vi "Read Multi Eval Meas Phase Error Results.vi"(8 "error in (no error)":errorcluster, 9 "Result Type (Current)":i32(ring) items=["Current"=0, "Average"=1, "Maximum"=4], 10 "Instance (1)":T1=1, 11 "VISA resource name":refnum<visa-resource-name>) -> (0 "error out":errorcluster, 1 "Phase Error Results":cluster{"Low":dbl, "High":dbl}[](array[cluster]) {"High" format="%^.3e"; "Low" format="%^.3e"}, 2 "Reliability":i32, 3 "VISA resource name out":refnum<visa-resource-name>)   [LabVIEW 2015, in "Rohde&Schwarz CMXP NR FR2 Measurement.lvlib"]
doc: "Starts a new single shot measurement and returns the multi eval measurement values of the phase error bar graphs for the OFDM symbols in the measured slot.\n\nAttributes:\nRSCMXPNRFR2M_ATTR_READ_MULTI_EVAL_MEASUREMENT_PERR_AVERAGE_RESULTS\nRSCMXPNRFR2M_ATTR_READ_MULTI_EVAL_MEASUREMENT_PERR_CURRENT_RESULTS\nRSCMXPNRFR2M_ATTR_READ_MULTI_EVAL_MEASUREMENT_PERR_MAXIMUM_RESULTS\n\nRemote-control commands:\nREAD:NRMMw:MEAS<i>:MEValuation:PERRor:AVERage?\nREAD:NRMMw:MEAS<i>:MEValuation:PERRor:CURRent?\nREAD:NRMMw:MEAS<i>:MEValuation:PERRor:MAXimum?"
uses:
  <instrlib>/Rohde&Schwarz CMXP NR FR2 Measurement/Rohde&Schwarz CMXP NR FR2 Measurement.lvlib
  <instrlib>/Rohde&Schwarz CMXP NR FR2 Measurement/Private/_Instance.ctl
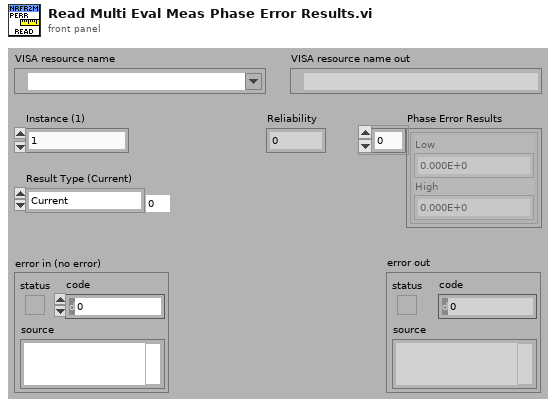
[diagram p1: front panel]
types:
  T1 = typedef "Rohde&Schwarz CMXP NR FR2 Measurement.lvlib/_Instance.ctl" = i32
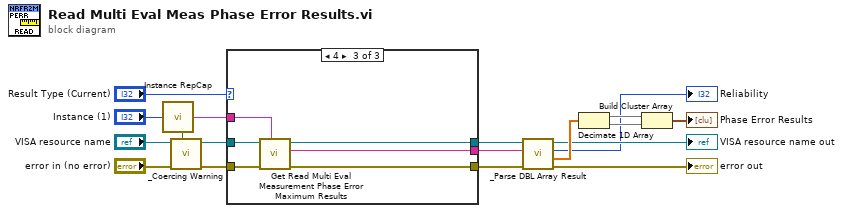
[diagram p0: block diagram]
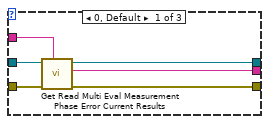
[diagram p2: hidden frame]
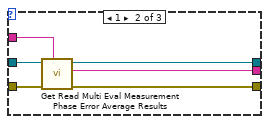
[diagram p3: hidden frame]
diagram:
  n1 = call <instrlib>:"Instance RepCap.vi"("Instance In"="Instance (1)") -> ("In Range?"=w3:bool, "RepCap Identifier Out"=w15:string)  [unwired: 1 in]
  n2 = call <instrlib>:"_Coercing Warning.vi"("In Range?"=w3, "error in (no error)"="error in (no error)", "VISA resource name"="VISA resource name") -> ("error out"=w4:errorcluster, "VISA resource name out"=w5:refnum<visa-resource-name>)  [unwired: 7 in]
  n3 = case shown="4" "Result Type (Current)" {
    tunnel: w4 -> [w24 w30 w36]
    tunnel: w5 -> [w23 w29 w35]
    tunnel: w15 -> [w22 w28 w34]
    tunnel: [w21 w27 w33] -> w13
    tunnel: [w20 w26 w32] -> w12
    tunnel: [w19 w25 w31] -> w14
    frame 0, Default {
      n4 = call "Get Read Multi Eval Measurement Phase Error Current Results"("Repeated Capabilities"=w22, "error in (no error)"=w24, "instrument handle"=w23) -> ("error out"=w21:errorcluster, "Read Multi Eval Measurement Phase Error Current Results"=w19:string, "instrument handle out"=w20:refnum<visa-resource-name>)  [unwired: 6 in]
    }
    frame 1 {
      n5 = call "Get Read Multi Eval Measurement Phase Error Average Results"("Repeated Capabilities"=w28, "error in (no error)"=w30, "instrument handle"=w29) -> ("error out"=w27:errorcluster, "Read Multi Eval Measurement Phase Error Average Results"=w25:string, "instrument handle out"=w26:refnum<visa-resource-name>)  [unwired: 6 in]
    }
    frame 4 {
      n6 = call "Get Read Multi Eval Measurement Phase Error Maximum Results"("Repeated Capabilities"=w34, "error in (no error)"=w36, "instrument handle"=w35) -> ("error out"=w33:errorcluster, "Read Multi Eval Measurement Phase Error Maximum Results"=w31:string, "instrument handle out"=w32:refnum<visa-resource-name>)  [unwired: 6 in]
    }
  }
  n7 = call <instrlib>:"_Parse DBL Array Result.vi"("error in (no error)"=w13, "Input String"=w14, "VISA resource name"=w12) -> ("error out"=→"error out":errorcluster, "Results"=w18:dbl[], "Reliability"=→"Reliability":i32, "VISA resource name out"=→"VISA resource name out":refnum<visa-resource-name>)  [unwired: 5 in]
  n8 = Decimate 1D Array(w18) -> (w17:dbl[], w16:dbl[])
  n9 = Build Cluster Array ("Index & Bundle Cluster Array")(w17, w16) -> (→"Phase Error Results":cluster{"Element":dbl, "Element":dbl}[])
